vi "Disconnected.vi"(8 "error in (no error)":errorcluster, 11 "SpectrumAnalyzerUI.lvclass":refnum<class "SpectrumAnalyzerUI.lvclass">) -> (0 "error out":errorcluster, 3 "SpectrumAnalyzerUI.lvclass":refnum<class "SpectrumAnalyzerUI.lvclass">)   [LabVIEW 2023, in "SpectrumAnalyzerUI.lvlib" / "SpectrumAnalyzerUI.lvclass"]
uses:
  SpectrumAnalyzerUI.lvclass
  SpectrumAnalyzerUI.lvclass/SpectrumAnalyzerUI.ctl
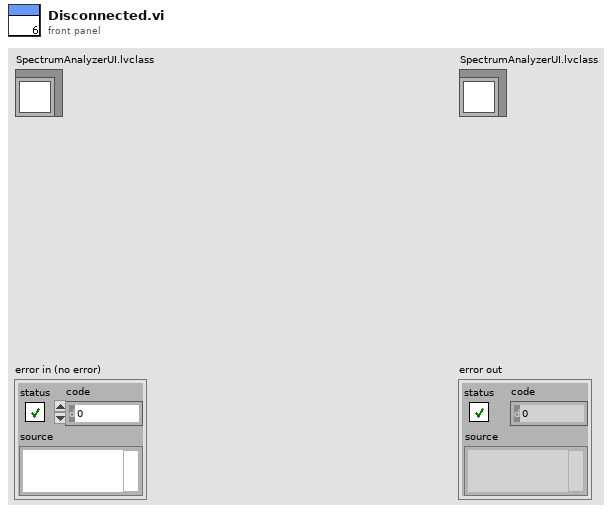
[diagram p1: front panel]
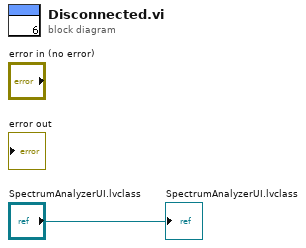
[diagram p0: block diagram]
diagram:
  "SpectrumAnalyzerUI.lvclass" <- "SpectrumAnalyzerUI.lvclass"
